vi "GNSS RF Test Get Default USL.vi"(8 "error in (no error)":errorcluster, 11 "Template Tx Test in":refnum<class "niDTS GNSS RF Test.lvclass">) -> (0 "error out":errorcluster, 2 "Default USL":T1, 3 "Template Tx Test out":refnum<class "niDTS GNSS RF Test.lvclass">)   [LabVIEW 2015, in "niDTS GNSS.lvlib" / "niDTS GNSS RF Test.lvclass"]
uses:
  niDTS GNSS RF Test.lvclass
  Includes/niDTS GNSS RF Test INC Results.ctl
  niDTS GNSS.lvlib
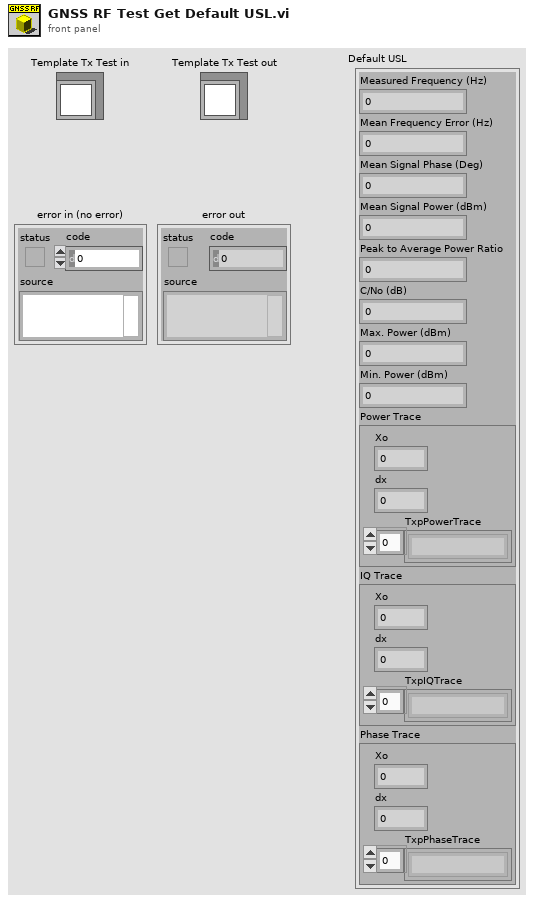
[diagram p1: front panel]
types:
  T1 = typedef "niDTS GNSS.lvlib/niDTS GNSS RF Test INC Results.ctl" = cluster{"Measured Frequency (Hz)":dbl, "Mean Frequency Error (Hz)":dbl, "Mean Signal Phase (Deg)":dbl, "Mean Signal Power (dBm)":dbl, "Peak to Average Power Ratio":dbl, "C/No (dB)":dbl, "Max. Power (dBm)":dbl, "Min. Power (dBm)":dbl, "Power Trace":cluster{"Xo":dbl, "dx":dbl, "TxpPowerTrace":string[]}, "IQ Trace":cluster{"Xo":dbl, "dx":dbl, "TxpIQTrace":string[]}, "Phase Trace":cluster{"Xo":dbl, "dx":dbl, "TxpPhaseTrace":string[]}}
  T2 = cluster{"Xo":dbl, "dx":dbl, "TxpPhaseTrace":string[]}
  T3 = cluster{"Xo":dbl, "dx":dbl, "TxpIQTrace":string[]}
  T4 = cluster{"Xo":dbl, "dx":dbl, "TxpPowerTrace":string[]}
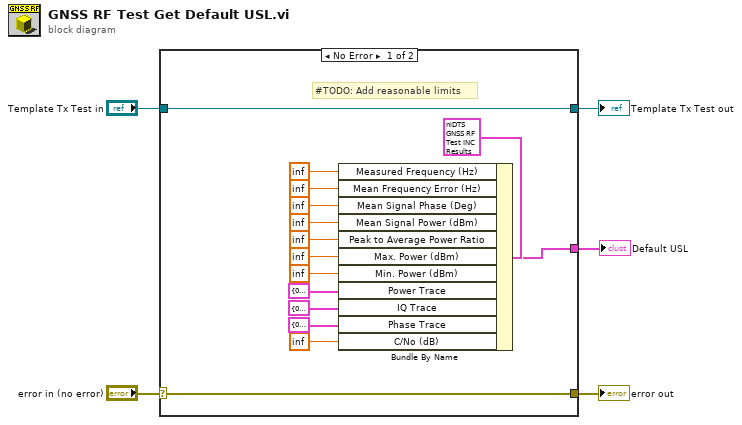
[diagram p0: block diagram]
diagram:
  n1 = case shown="No Error" "error in (no error)" {
    selector: "error in (no error)" -> [w20 w22]
    tunnel: [w20 w22] -> w4
    tunnel: [w19 w21] -> w2
    tunnel: "Template Tx Test in" -> [w19 w21]
    tunnel: [w17 _] -> w1
    frame No Error {
      # "#TODO: Add reasonable limits"
      n2 = Bundle By Name(cluster=T1 {"Measured Frequency (Hz)"=0.0, "Mean Frequency Error (Hz)"=0.0, "Mean Signal Phase (Deg)"=0.0, "Mean Signal Power (dBm)"=0.0, "Peak to Average Power Ratio"=0.0, "C/No (dB)"=0.0, "Max. Power (dBm)"=0.0, "Min. Power (dBm)"=0.0, "Power Trace"={"Xo"=0.0, "dx"=0.0, "TxpPowerTrace"=[]}, "IQ Trace"={"Xo"=0.0, "dx"=0.0, "TxpIQTrace"=[]}, "Phase Trace"={"Xo"=0.0, "dx"=0.0, "TxpPhaseTrace"=[]}} ("Default LSL"), "Measured Frequency (Hz)"=inf ("Measured Frequency"), "Mean Frequency Error (Hz)"=inf ("Mean Frequency Error"), "Mean Signal Phase (Deg)"=inf ("Mean Phase"), "Mean Signal Power (dBm)"=inf ("Mean Power"), "Peak to Average Power Ratio"=inf ("Peak to Average Power Ratio (PAPR)"), "Max. Power (dBm)"=inf ("Max. Power"), "Min. Power (dBm)"=inf ("Min. Power"), "Power Trace"=T4 {"Xo"=0.0, "dx"=0.0, "TxpPowerTrace"=[]}, "IQ Trace"=T3 {"Xo"=0.0, "dx"=0.0, "TxpIQTrace"=[]}, "Phase Trace"=T2 {"Xo"=0.0, "dx"=0.0, "TxpPhaseTrace"=[]}, "C/No (dB)"=inf) -> (w17:T1)
    }
    frame Error {
    }
  }
  "error out" <- w4
  "Template Tx Test out" <- w2
  "Default USL" <- w1
